vi "Close (Resources).vi"(8 "error in (no error)":errorcluster, 11 "Resources in":refnum<k20>[](array[refnum])) -> (0 "error out":errorcluster)   [LabVIEW 2014, in "nisyscfg.lvlib"]
doc: "Closes references to multiple hardware resources."
uses:
  nisyscfg.lvlib
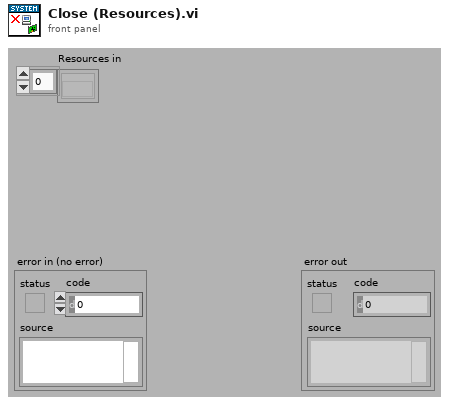
[diagram p1: front panel]
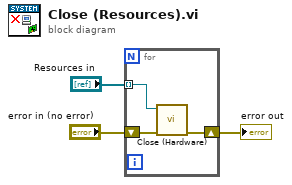
[diagram p0: block diagram]
diagram:
  n1 = for {
    tunnel: "Resources in" -> [w6] mode=indexing
    shift-right: [w4] -> w1
    shift-left: "error in (no error)" -> [w5]
    n2 = call "Close (Hardware).vi"("error in (no error)"=w5, "Resource in"=w6) -> ("error out"=w4:errorcluster)  [unwired: 9 in]
  }
  "error out" <- w1
